vi "Day6-1.vi"() -> ()   [LabVIEW 2020]
panel:
  out "x+1":i32
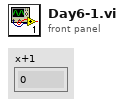
[diagram p1: front panel]
diagram:
  w4 = 14
  n1 = String To Byte Array(string="qzbzwwghwhwdhdqhhbhfbfsstggdsssgzgdzzdbbbzmbzzvlldppjnjlltwtsszwswgssjnsjnnfqfzqqjzjfjmfmwfmfhfnnmdnmnllbzzlbzlzflldzdbzbsbdddpgdppzhphhjjtccjgcgrgjgcjgjjsbjbffsgsqqrsqqgppgmgcmmrdrqdqbqmmctchcgcdgdwdwcdcjcfjccmpmlpllqqpmpllhfhchppwwdmdhdphpvprrhwhgwwlrwlwggwlwqqnmqnqrrbbzdzwddqzznllzwlljsscqqtlltppqspswsttlrttnvvvwllfslsjsfjssnqnbbbvgvlltjtltjljmljjfgfbggcbgbmbjjvwjvjgvgzvvzddrjdddrwrlrlgldlhlwwcddbsbbtwwcssrnndvvsbsnbsbmbnmngnpgpphfhzhshllltqtppnrrzpzrpzzrttmbmssbrbmbsmsnspnsncscwwmjwmwdmwmrmvmqvqvjqvvnrrtntwwwwsrwrnwnrwwwlslrlhrllvpvhppdpprrgzrgzggqmqgmgvghhsmhhjljfflrflfrlrzzbjjqmmmcncddvh...") -> (unsigned byte array=w6:u8[])
  n2 = Index Array(array=w6) -> (element=w5:u8)  [unwired: 1 in]
  n3 = Initialize Array(w5, w4) -> (w3:u8[])
  n4 = for {
    tunnel: w6 -> [w15] mode=indexing
    tunnel: w4 -> [w10]
    shift-right: [w13] -> _
    shift-left: w3 -> [w17]
    tunnel: [w8] -> w2
    i -> [w8]
    stop <- w9 stop-if-true
    w14 = set{u8} {}  # Size: 0
    n5 = Quotient & Remainder(x=w8, y=w10) -> (x-y*floor(x/y)=w16:i32)  [unwired: 1 out]
    n6 = Replace Array Subset(array=w17, new element=w15, index=w16) -> (w13:u8[])
    n7 = for {
      shift-right: [w18] -> w12
      shift-left: w14 -> [w20]
      tunnel: w13 -> [w19] mode=indexing
      n8 = Insert Into Set(10:w19, 11:w20) -> (3:w18:set{u8})  [unwired: 1 out]
    }
    n9 = Collection Size(1:w12) -> (0:w11:i32)
    n10 = Greater Or Equal?(x=w11, y=w10) -> (x >= y?=w9:bool)
  }
  n11 = Increment(x=w2) -> (x+1=→"x+1":i32)
